vi "Read State Update Rate.vi"(8 "error in (no error)":errorcluster, 11 "RDS State Tracker in":refnum<class "RDS State Tracker.lvclass">) -> (0 "error out":errorcluster, 2 "State Update Rate":dbl, 3 "RDS State Tracker out":refnum<class "RDS State Tracker.lvclass">)   [LabVIEW 2015, in "RDS State Tracker.lvlib" / "RDS State Tracker.lvclass"]
uses:
  RDS State Tracker.lvclass
  RDS State Tracker.lvclass/RDS State Tracker.ctl
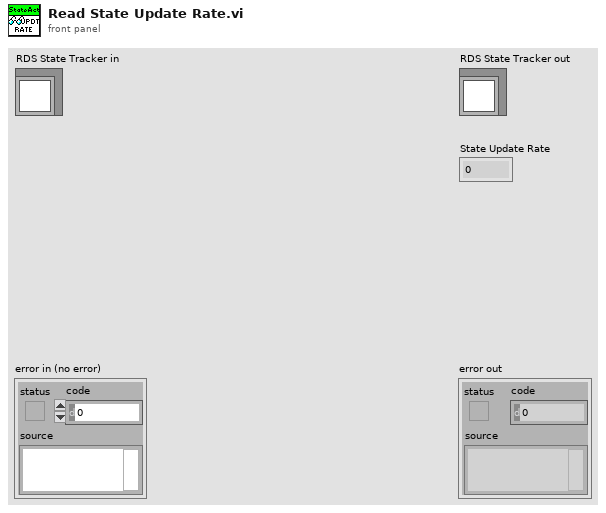
[diagram p1: front panel]
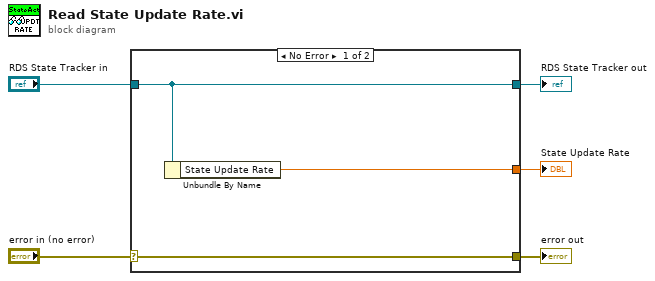
[diagram p0: block diagram]
diagram:
  n1 = case shown="No Error" "error in (no error)" {
    selector: "error in (no error)" -> [w8 w9]
    tunnel: [w8 w9] -> w4
    tunnel: [w7 w10] -> w2
    tunnel: "RDS State Tracker in" -> [w7 w10]
    tunnel: [w6 _] -> w1
    frame No Error {
      n2 = Unbundle By Name(w7) -> ("State Update Rate"=w6:dbl)
    }
    frame Error {
    }
  }
  "error out" <- w4
  "RDS State Tracker out" <- w2
  "State Update Rate" <- w1
